vi "General_Remove Dup 1D Array (U32).vi"(8 "Error In (no Error)":errorcluster, 11 "Color Array":u32[](array[colorbox])) -> (0 "Error Out":errorcluster, 2 "Indices Of Removed Elements Out":i32[](array[numeric]), 3 "Color Array Out":u32[](array[colorbox]))   [LabVIEW 2009]
doc: "Modified OpenG Vi to remove all duplicate colors"
panel:
  # "Remove Duplicates from 1D Array.vi\n\nRemoves duplicate array elements and returns the indices of the removed elements\n\nPlease visit http://www.OpenG.org to learn about the\nOpen Source LabVIEW software movement.\n\nNOTICE -- YOU MUST LEAVE THIS NOTICE IN PLACE.  PER THE TERMS OF THE LICENSE BELOW, YOU MAY SUBLICENSE THIS SOFTWARE \nIN ANY WAY THAT DOES NOT CONFLICT WITH THIS LICENSE.\n\n### BSD License (http://www.opensource.org/licenses/bsd-license.php) Begin ###\n \nCopyright (c) 2002, Jim Kring <jim@jimkring.com>\n\nAll rights reserved.\n\nRedistribution and use in source and binary forms, with or without modification, are permitted provided that the following conditions are met:\n\n    * Redistributions of source code must retain the above copyright notice, this list of conditions and the following disclaimer.\n    * Redistributions in binary form must reproduce the above copyright notice, this list of conditions and the following disclaimer in the \n       documentation and/or other materials provided with the distribution.\n    * Neither the name of SciWare, James Kring, Inc., nor the names of its contributors may be used to endorse or promote products derived \n       from this software without specific prior written permission.\n\nTHIS SOFTWARE IS PROVIDED BY THE COPYRIGHT HOLDERS AND CONTRIBUTORS \"AS IS\" AND ANY EXPRESS OR IMPLIED WARRANTIES, \nINCLUDING, BUT NOT LIMITED TO, THE IMPLIED WARRANTIES OF MERCHANTABILITY AND FITNESS FOR A PARTICULAR PURPOSE ARE \nDISCLAIMED. IN NO EVENT SHALL THE COPYRIGHT OWNER OR CONTRIBUTORS BE LIABLE FOR ANY DIRECT, INDIRECT, INCIDENTAL,\n SPECIAL, EXEMPLARY, OR CONSEQUENTIAL DAMAGES (INCLUDING, BUT NOT LIMITED TO, PROCUREMENT OF SUBSTITUTE GOODS OR \nSERVICES; LOSS OF USE, DATA, OR PROFITS; OR BUSINESS INTERRUPTION) HOWEVER CAUSED AND ON ANY THEORY OF LIABILITY, \nWHETHER IN CONTRACT, STRICT LIABILITY, OR TORT (INCLUDING NEGLIGENCE OR OTHERWISE) ARISING IN ANY WAY OUT OF THE USE \nOF THIS SOFTWARE, EVEN IF ADVISED OF THE POSSIBILITY OF SUCH DAMAGE.\n\n### BSD License End ###"
  # "[OpenG VI Tags] ***Do Not Remove***\nSVN Revision = 593\nSVN Revision Date = 2006-12-19 19:10:48 -0800 (Tue, 19 Dec 2006)\nPackage = oglib_array-2.7-1\nDepends ="
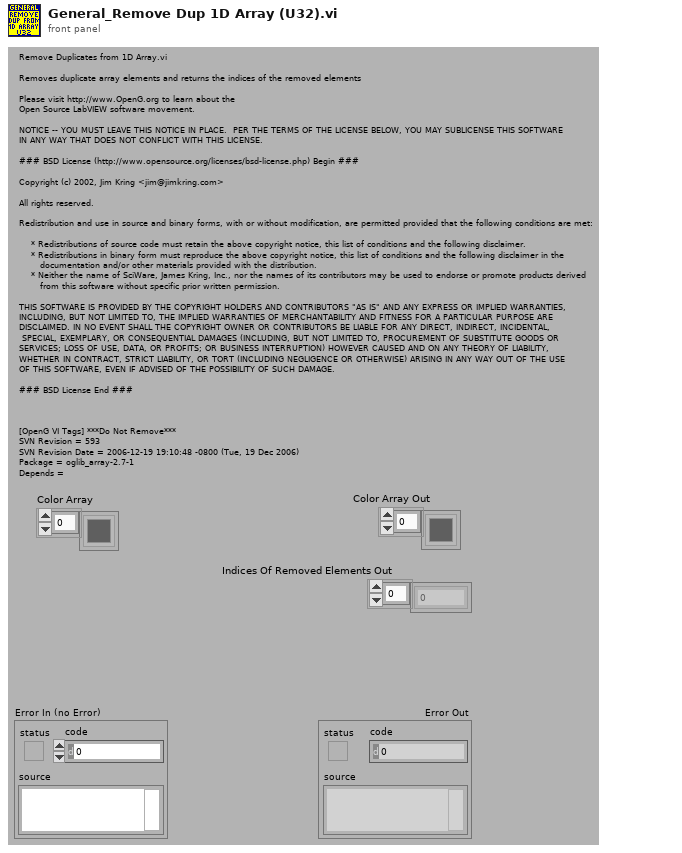
[diagram p1: front panel]
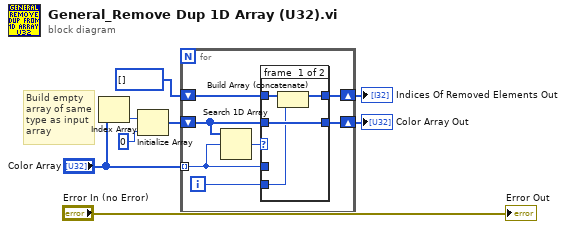
[diagram p0: block diagram]
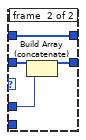
[diagram p2: hidden frame]
diagram:
  # "Build empty array of same type as input array"
  n1 = Index Array(array="Color Array") -> (element=w4:u32)  [unwired: 1 in]
  n2 = Initialize Array(w4, 0 ("Dimension Size")) -> (w3:u32[])
  n3 = for {
    tunnel: "Color Array" -> [w14] mode=indexing
    shift-right: [w13] -> w7
    shift-left: w3 -> [w12]
    shift-right: [w10] -> w5
    shift-left: i32[] [] -> [w9]
    i -> [w11]
    n4 = Search 1D Array(1D array=w12, element=w14) -> (index of element=w15:i32)  [unwired: 1 in]
    n5 = case shown="Default" w15 {
      tunnel: w14 -> [_ w23]
      tunnel: [w19 w21] -> w13
      tunnel: w12 -> [w19 w22]
      tunnel: w11 -> [w16 _]
      tunnel: [w17 w20] -> w10
      tunnel: w9 -> [w18 w20]
      frame #0 {
        n6 = Build Array (concatenate)(w18, w16) -> (w17:i32[])
      }
      frame #1 {
        n7 = Build Array (concatenate)(w22, w23) -> (w21:u32[])
      }
    }
  }
  "Color Array Out" <- w7
  "Indices Of Removed Elements Out" <- w5
  "Error Out" <- "Error In (no Error)"
